vi "TEST - Array to Map - Map to Array.vi"(8 "error in":errorcluster) -> (0 "error out":errorcluster, 2 "Pass?":bool)   [LabVIEW 2020, in "test_openg_array.lvlib"]
uses:
  test_openg_array.lvlib
  source/library/Get Collection Subtype.vi
  <vilib>/addons/_JKI Toolkits/Caraya/classes/Assert/Assert True.vi
  <vilib>/addons/_JKI Toolkits/Caraya/classes/Test/Test.lvclass
  <vilib>/addons/_JKI Toolkits/Caraya/classes/Assert/Assert.lvclass
  source/library/openg_variant.lvlib
panel:
  out "Pass (Map to Array -> Array to Map)?":bool
  out "Pass (Set to MAP)?":bool
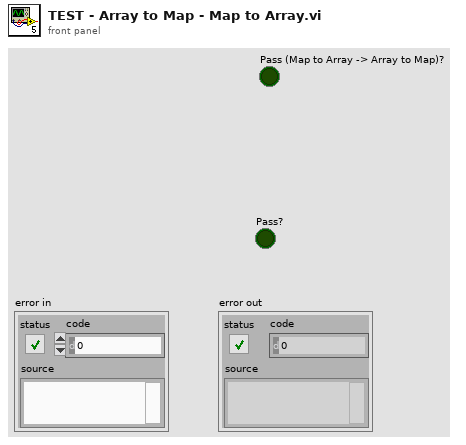
[diagram p1: front panel]
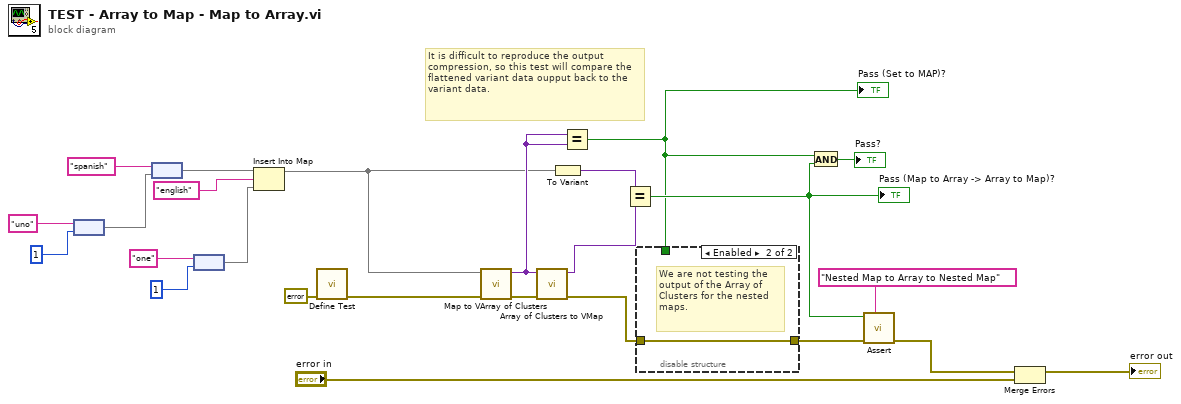
[diagram p0: block diagram]
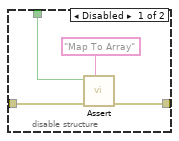
[diagram p2: hidden frame]
diagram:
  # "It is difficult to reproduce the output compression, so this test will compare the flattened variant data oupput back to the variant data."
  n1 = node("uno" ("key"), 1) -> (w7:map{string, i32})
  n2 = node("spanish" ("key"), w7) -> (w6:map{string, map{string, i32}})
  n3 = node("one" ("key"), 1) -> (w2:map{string, i32})
  n4 = Insert Into Map(map in=w6, key="english", value=w2) -> (map out=w1:map{string, map{string, i32}})  [unwired: 2 out]
  n5 = call <vilib>:"Define Test.vi"("error in (no error)"=errorcluster {"status"=FALSE, "code"=0, "source"=""}) -> ("error out"=w17:errorcluster)  [unwired: 9 in, 1 out]
  n6 = call "Map to VArray of Clusters.vi"("error in"=w17, "Map"=w1) -> ("error out"=w16:errorcluster, "Array of Clusters (key-value)"=w12:variant)  [unwired: 8 in]
  n7 = call "Array of Clusters to VMap.vi"("error in"=w16, "Array of Clusters (key-value)"=w12) -> ("error out"=w15:errorcluster, "Map"=w14:variant)  [unwired: 8 in]
  n8 = To Variant(anything=w1) -> (Variant=w25:variant)
  n9 = Equal?(x=w12, y=w12) -> (x = y?=w11:bool)
  "Pass (Set to MAP)?" <- w11
  n10 = Equal?(x=w25, y=w14) -> (x = y?=w22:bool)
  "Pass (Map to Array -> Array to Map)?" <- w22
  n11 = disable-structure shown="Enabled" {
    disable-tunnel: w15 -> [w29 w30]
    disable-tunnel: [w28 w30] -> w13
    disable-tunnel: w11 -> [w26 _]
    frame Disabled {
      n12 = call-poly <vilib>:"Assert.vi"("Label"="Map To Array" ("Label (VI Title)"), "error in (no error)"=w29, "True?"=w26) -> ("error out"=w28:errorcluster)  [unwired: 7 in, 1 out]
    }
    frame Enabled {
      # "We are not testing the output of the Array of Clusters for the nested maps."
    }
  }
  n13 = And(x=w11, y=w22) -> (x .and. y?=→"Pass?":bool)
  n14 = call-poly <vilib>:"Assert.vi"("Label"="Nested Map to Array to Nested Map" ("Label (VI Title)"), "error in (no error)"=w13, "True?"=w22) -> ("error out"=w18:errorcluster)  [unwired: 7 in, 1 out]
  n15 = Merge Errors(w18, "error in") -> (→"error out":errorcluster)
